vi "read_write.vi"(5 "Query?":bool, 6 "error in":errorcluster, 8 "Command":string, 9 "VISA handle in":refnum<visa-resource-name>) -> (0 "error out":errorcluster, 2 "Response":string, 3 "VISA handle out":refnum<visa-resource-name>, 4 "TimeoutFlag":bool)   [LabVIEW 2011]
doc: "This VI allows to send a command to the controller SMC 100 and to receive a response via the connection RS232. It is used in each VI."
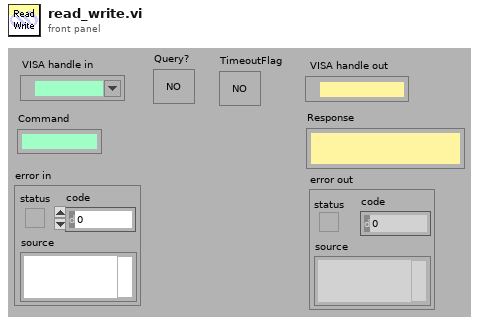
[diagram p1: front panel]
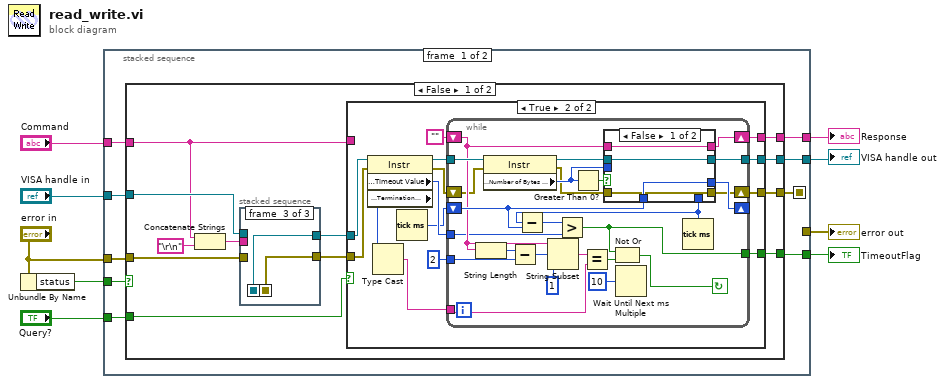
[diagram p0: block diagram]
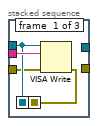
[diagram p2: hidden frame]
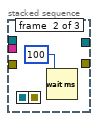
[diagram p3: hidden frame]
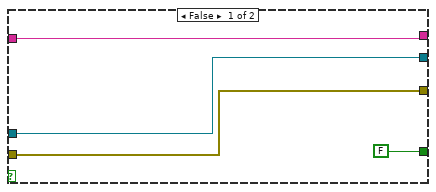
[diagram p4: hidden frame]
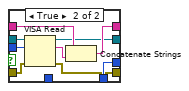
[diagram p5: hidden frame]
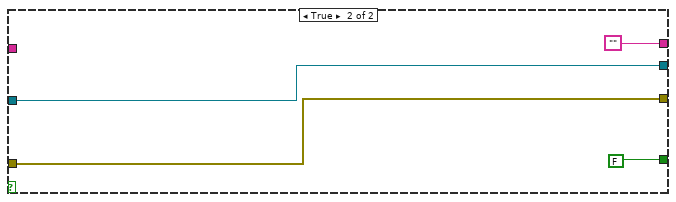
[diagram p6: hidden frame]
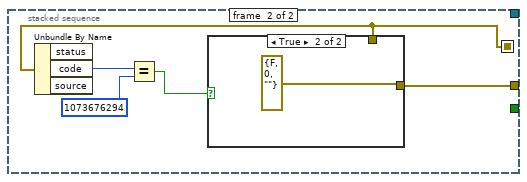
[diagram p7: hidden frame]
diagram:
  n1 = Unbundle By Name("error in") -> ("status"=w7:bool)
  n2 = stacked-sequence {
    seq-local: [w14 _] -> [_ w98]
    tunnel: "VISA handle in" -> [w18 _]
    tunnel: [_ w99] -> w8
    tunnel: w7 -> [w17 _]
    tunnel: "error in" -> [w16 _]
    tunnel: "Query?" -> [w15 _]
    tunnel: "Command" -> [w13 _]
    tunnel: [w12 _] -> w1
    tunnel: [w11 _] -> w3
    tunnel: [w10 _] -> w2
    frame #0 {
      n3 = case shown="False" w17 {
        tunnel: w18 -> [w30 w97]
        tunnel: [w26 w97] -> w12
        tunnel: [w25 w96] -> w14
        tunnel: w16 -> [w29 w96]
        tunnel: [w24 ""] -> w10
        tunnel: [w23 FALSE] -> w11
        tunnel: w15 -> [w20 _]
        tunnel: w13 -> [w19 _]
        frame False {
          n4 = Concatenate Strings(w19, "\r\n") -> (w21:string)
          n5 = stacked-sequence {
            seq-local: [w33 _ _] -> [_ _ w37]
            seq-local: [w31 _ _] -> [_ _ w36]
            tunnel: w30 -> [w33 _ _]
            tunnel: w21 -> [w34 _ _]
            tunnel: w29 -> [w32 _ _]
            tunnel: [_ _ w37] -> w28
            tunnel: [_ _ w36] -> w27
            frame #0 {
              n6 = VISA Write(VISA resource name=w33, write buffer=w34, error in (no error)=w32) -> (error out=w31:errorcluster)  [unwired: 2 out]
            }
            frame #1 {
              n7 = Wait (ms)(milliseconds to wait=u32 100 ("Delay (ms)")) -> ()  [unwired: 1 out]
            }
            frame #2 {
            }
          }
          n8 = case shown="True" w20 {
            tunnel: [w40 w42] -> w25
            tunnel: [w41 w47] -> w26
            tunnel: w28 -> [w41 w55]
            tunnel: w27 -> [w40 w54]
            tunnel: [w38 w46] -> w24
            tunnel: [FALSE w44] -> w23
            tunnel: w19 -> [w38 _]
            frame False {
            }
            frame True {
              n9 = property class="Instr"(reference=w55, error in=w54) -> (reference out=w53:refnum<visa-resource-name>, error out=w52:errorcluster, "General Settings:Timeout Value"=w51:u32, "Message Based Settings:Termination Character"=w50:u8)
              n10 = Type Cast(x=w50) -> (*(type *) &x=w48:string)  [unwired: 1 in]
              n11 = Tick Count (ms)() -> (millisecond timer value=w49:u32)
              n12 = while {
                tunnel: 2 -> [w58]
                tunnel: w51 -> [w66]
                tunnel: w53 -> [w80]
                shift-right: [w76] -> w46
                shift-left: "" -> [w67]
                shift-right: [w74] -> _
                shift-left: w49 -> [w73]
                tunnel: w48 -> [w68]
                tunnel: [w63] -> w44
                tunnel: [w62] -> w47
                shift-right: [w56] -> w42
                shift-left: w52 -> [w61]
                stop <- w64 continue-if-true
                n13 = String Length(string=w67) -> (length=w71:i32)
                n14 = property class="Instr"(reference=w80, error in=w61) -> (reference out=w78:refnum<visa-resource-name>, error out=w59:errorcluster, "Serial Settings:Number of Bytes at Serial Port"=w77:u32)
                n15 = Subtract(x=w71, y=w58) -> (x-y=w70:i32)
                n16 = String Subset(string=w67, offset (0)=w70, length (rest)=1 ("longueur (reste)")) -> (substring=w69:string)
                n17 = Greater Than 0?(x=w77) -> (x > 0?=w79:bool)
                n18 = Equal?(x=w69, y=w68) -> (x = y?=w65:bool)
                n19 = Wait Until Next ms Multiple(millisecond multiple=u32 10) -> ()  [unwired: 1 out]
                n20 = Tick Count (ms)() -> (millisecond timer value=w75:u32)
                n21 = Subtract(x=w75, y=w73) -> (x-y=w72:u32)
                n22 = Greater?(x=w72, y=w66) -> (0:w63:bool)
                n23 = case shown="False" w79 {
                  tunnel: w78 -> [w82 w93]
                  tunnel: w77 -> [_ w92]
                  tunnel: w67 -> [w84 w90]
                  tunnel: [w84 w89] -> w76
                  tunnel: w75 -> [_ w88]
                  tunnel: [w83 w88] -> w74
                  tunnel: w73 -> [w83 _]
                  tunnel: [w82 w87] -> w62
                  tunnel: w59 -> [w81 w86]
                  tunnel: [w81 w85] -> w56
                  frame False {
                  }
                  frame True {
                    n24 = VISA Read(VISA resource name=w93, byte count=w92, error in (no error)=w86) -> (VISA resource name out=w87:refnum<visa-resource-name>, read buffer=w91:string, error out=w85:errorcluster)  [unwired: 1 out]
                    n25 = Concatenate Strings(w90, w91) -> (w89:string)
                  }
                }
                n26 = Not Or(1:w65, 2:w63) -> (0:w64:bool)
              }
            }
          }
        }
        frame True {
        }
      }
    }
    frame #1 {
      n27 = Unbundle By Name(w98) -> ("code"=w102:i32)  [unwired: 2 out]
      n28 = Equal?(x=w102, y=1073676294) -> (x = y?=w101:bool)
      n29 = case shown="True" w101 {
        tunnel: w98 -> [w103 _]
        tunnel: [w103 errorcluster {"status"=FALSE, "code"=0, "source"=""} ("sortie d'erreur 2")] -> w99
        frame False {
        }
        frame True {
        }
      }
    }
  }
  "VISA handle out" <- w1
  "error out" <- w8
  "Response" <- w2
  "TimeoutFlag" <- w3
